vi "jitterGraph.vi"(8 "Y-jitter":dbl, 9 "X-jitter":dbl, 11 "GraphPlots":cluster{"Array":dbl[], "Array":dbl[]}[](array[cluster])) -> (3 "jitteredGraphPlots":cluster{"Array":dbl[], "Array":dbl[]}[](array[cluster]))   [LabVIEW 2013]
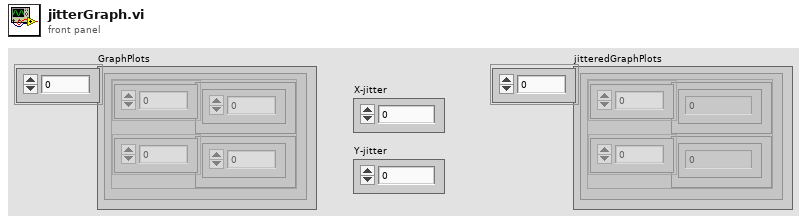
[diagram p1: front panel]
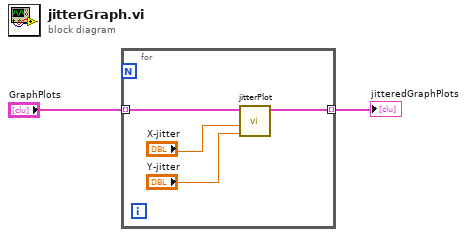
[diagram p0: block diagram]
diagram:
  n1 = for {
    tunnel: "GraphPlots" -> [w4] mode=indexing
    tunnel: [w3] -> w1 mode=indexing
    n2 = call "jitterPlot.vi"("Y-jitter"="Y-jitter", "X-jitter"="X-jitter", "PlotCluster"=w4) -> ("JitteredPlotCluster"=w3:cluster{"X":dbl[], "Y":dbl[]})  [unwired: 8 in]
  }
  "jitteredGraphPlots" <- w1
